vi "Kalman.vi"(2 "szigmaw":dbl, 3 "szigmav":dbl, 4 "Pk-1|k-1":dbl, 5 "Zetak-1|k-1":dbl, 6 "uk":dbl, 7 "zk":dbl) -> (0 "Zetak|k":dbl, 1 "Pk|k":dbl)   [LabVIEW 2011]
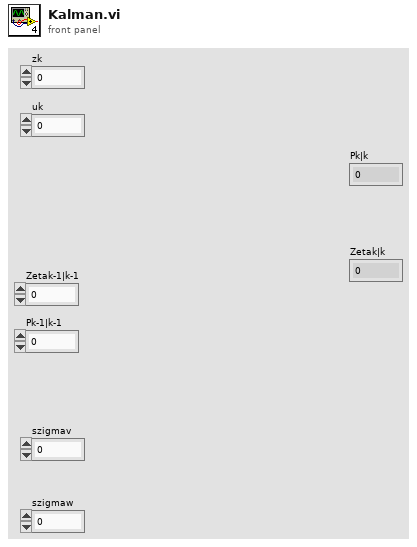
[diagram p1: front panel]
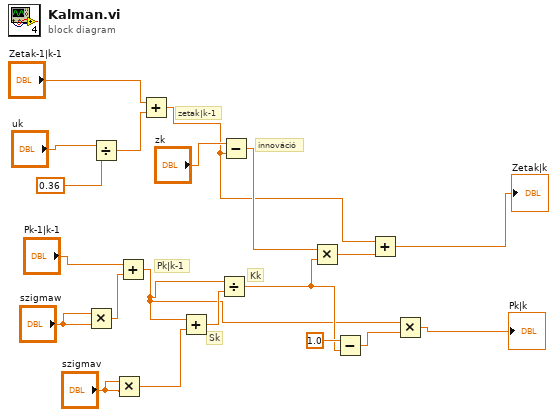
[diagram p0: block diagram]
diagram:
  # "Kk"
  # "Sk"
  # "innováció"
  # "Pk|k-1"
  # "zetak|k-1"
  n1 = Multiply(x="szigmaw", y="szigmaw") -> (x*y=w15:dbl)
  n2 = Divide(x="uk", y=0.36) -> (x/y=w20:dbl)
  n3 = Multiply(x="szigmav", y="szigmav") -> (x*y=w11:dbl)
  n4 = Add(x="Pk-1|k-1", y=w15) -> (x+y=w2:dbl)
  n5 = Add(x="Zetak-1|k-1", y=w20) -> (x+y=w8:dbl)
  n6 = Add(x=w2, y=w11) -> (x+y=w10:dbl)
  n7 = Divide(x=w2, y=w10) -> (x/y=w4:dbl)
  n8 = Subtract(x="zk", y=w8) -> (x-y=w9:dbl)
  n9 = Multiply(x=w9, y=w4) -> (x*y=w7:dbl)
  n10 = Subtract(x=1.0, y=w4) -> (x-y=w3:dbl)
  n11 = Add(x=w8, y=w7) -> (x+y=→"Zetak|k":dbl)
  n12 = Multiply(x=w2, y=w3) -> (x*y=→"Pk|k":dbl)
